vi "Redetection_Baseline calculation.vi"(6 "Sweep #":i32, 8 "File Paramters":T2, 9 "Sweep trace (1D)":cluster{"Ramp Pattern":dbl[], "X":dbl[]}[](array[cluster]), 10 "Detected event":cluster{dbl[][]}, 11 "Data type":T4 items=["AXON", "HEKA"]) -> (3 "New baseline info":cluster{dbl[][]})   [LabVIEW 2017]
uses:
  Data type_new.ctl
  Baseline selection.ctl
  <vilib>/Analysis/baseanly.llb/Mean (DBL).vi
  <vilib>/Analysis/NI_AALBase.lvlib
  <vilib>/Analysis/NI_AALPro.lvlib
panel:
  out "Baseline":cluster{T1[], dbl[]}
  out "XY 그래프":cluster{dbl[], dbl[]}[](graph)
  out "Histogram Graph":T3(graph) caption="히스토그램 그래프"
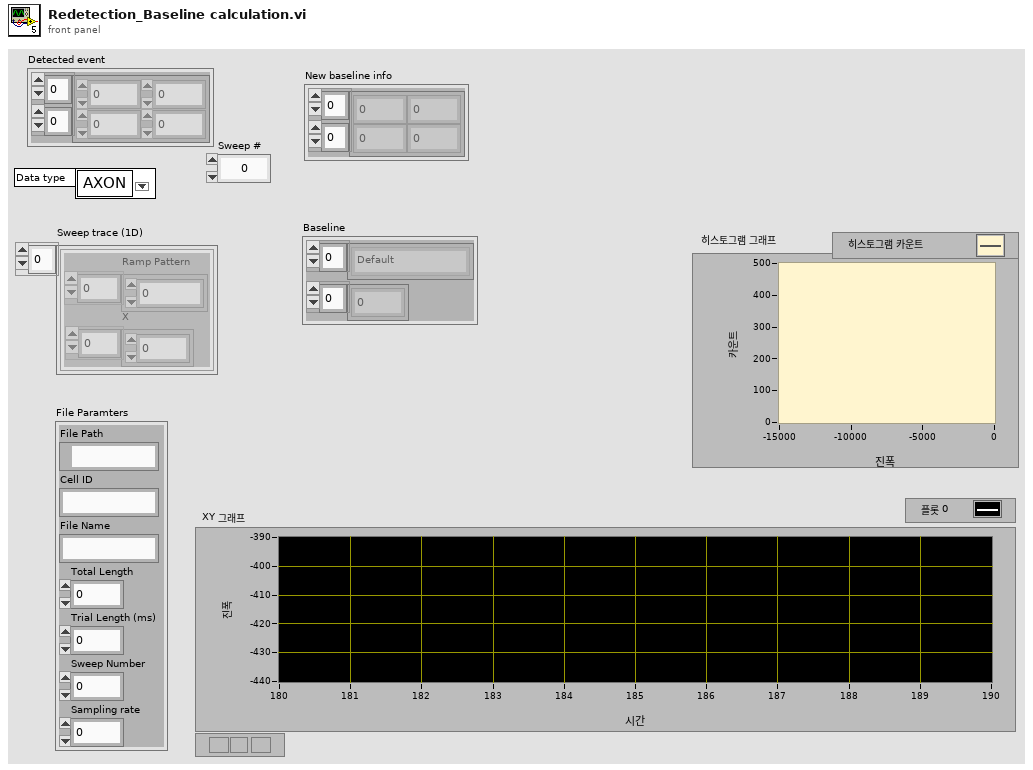
[diagram p1: front panel]
types:
  T1 = typedef "Baseline selection.ctl" = enum16{"Default", "Manual"}
  T2 = cluster{"File Path":path, "Cell ID":string, "File Name":string, "Total Length":i32, "Trial Length (ms)":dbl, "Sweep Number":dbl, "Sampling rate":dbl}
  T3 = cluster{"X Values":dbl[], "Histogram: h(x)":i32[]}
  T4 = typedef "Data type_new.ctl" = u16
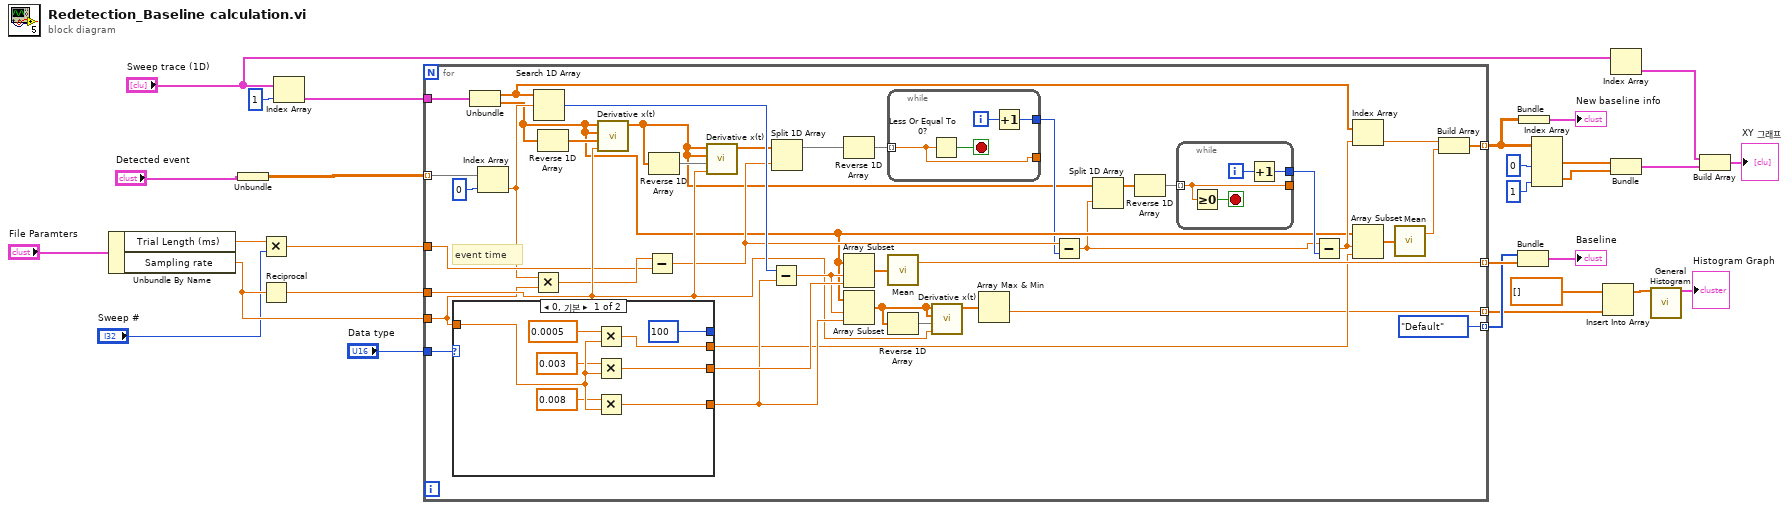
[diagram p0: block diagram]
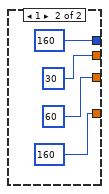
[diagram p2: hidden frame]
diagram:
  n1 = Unbundle By Name("File Paramters") -> ("Trial Length (ms)"=w18:dbl, "Sampling rate"=w4:dbl)
  n2 = Unbundle("Detected event") -> (w1:dbl[][])
  n3 = Multiply(x=w18, y="Sweep #") -> (x*y=w5:dbl)
  n4 = Reciprocal(x=w4) -> (1/x=w11:dbl)
  n5 = Index Array(array="Sweep trace (1D)", index=1 ("인덱스")) -> (element=w15:cluster{"Ramp Pattern":dbl[], "X":dbl[]})
  n6 = for {
    tunnel: w15 -> [w41]
    tunnel: w1 -> [w43] mode=indexing
    tunnel: [w66] -> w14 mode=indexing
    tunnel: "Data type" -> [w68]
    tunnel: [Baseline_selection."Default" ("Baseline selection")] -> w13 mode=indexing
    tunnel: w11 -> [w40]
    tunnel: [w53] -> w10 mode=indexing
    tunnel: [w52] -> w12 mode=indexing
    tunnel: w4 -> [w35]
    tunnel: w5 -> [w38]
    # "event time"
    n7 = case shown="0, 기본" w68 {
      tunnel: [w78 160 ("y")] -> w56
      tunnel: [100 ("길이") 160 ("길이")] -> _
      tunnel: [w79 60 ("길이")] -> w65
      tunnel: [w77 30 ("길이")] -> w55
      tunnel: w35 -> [w83 _]
      frame 0, Default {
        n8 = Multiply(x=0.0005, y=w83) -> (x*y=w77:dbl)
        n9 = Multiply(x=0.003, y=w83) -> (x*y=w79:dbl)
        n10 = Multiply(x=0.008, y=w83) -> (x*y=w78:dbl)
      }
      frame 1 {
      }
    }
    n11 = Unbundle(w41) -> ("Ramp Pattern"=w37:dbl[], "X"=w33:dbl[])
    n12 = Index Array(array=w43, index=0 ("인덱스")) -> (element=w36:dbl)
    n13 = Multiply(x=w36, y=w35) -> (x*y=w39:dbl)
    n14 = Search 1D Array(1D array=w37, element=w36) -> (index of element=w63:i32)  [unwired: 1 in]
    n15 = Reverse 1D Array(array=w33) -> (reversed array=w49:dbl[])
    n16 = call <vilib>:"Derivative x(t).vi"("dt"=w40, "Final Condition"=w49, "Initial Condition"=w33, "X"=w33) -> ("dX/dt"=w29:dbl[])  [unwired: 6 in, 1 out]
    n17 = Subtract(x=w39, y=w38) -> (x-y=w34:dbl)
    n18 = Reverse 1D Array(array=w29) -> (reversed array=w48:dbl[])
    n19 = call <vilib>:"Derivative x(t).vi"("dt"=w40, "Final Condition"=w48, "Initial Condition"=w29, "X"=w29) -> ("dX/dt"=w32:dbl[])  [unwired: 6 in, 1 out]
    n20 = Subtract(x=w63, y=w56) -> (x-y=w54:dbl)
    n21 = Split 1D Array(array=w32, index=w34) -> (first subarray=w47:dbl[])  [unwired: 1 out]
    n22 = Reverse 1D Array(array=w47) -> (reversed array=w46:dbl[])
    n23 = Array Subset(array=w33, index=w54, length=w65) -> (w64:dbl[])
    n24 = Array Subset(array=w33, index=w54, length=w56) -> (w62:dbl[])
    n25 = while {
      tunnel: w46 -> [w71] mode=indexing
      tunnel: [w71] -> _
      tunnel: [w69] -> w31
      i -> [w70]
      stop <- w72 stop-if-true
      n26 = Less Or Equal To 0?(x=w71) -> (x <= 0?=w72:bool)
      n27 = Increment(x=w70) -> (x+1=w69:i32)
    }
    n28 = call-poly <vilib>:"Mean.vi"("X"=w64) -> ("mean"=w66:dbl)  [unwired: 1 out]
    n29 = Reverse 1D Array(array=w62) -> (reversed array=w57:dbl[])
    n30 = call <vilib>:"Derivative x(t).vi"("dt"=w40, "Final Condition"=w57, "Initial Condition"=w62, "X"=w62) -> ("dX/dt"=w51:dbl[])  [unwired: 6 in, 1 out]
    n31 = Array Max & Min(array=w51) -> (min value=w52:dbl)  [unwired: 3 out]
    n32 = Subtract(x=w34, y=w31) -> (x-y=w30:dbl)
    n33 = Split 1D Array(array=w29, index=w30) -> (first subarray=w50:dbl[])  [unwired: 1 out]
    n34 = Reverse 1D Array(array=w50) -> (reversed array=w58:dbl[])
    n35 = while {
      tunnel: w58 -> [w75] mode=indexing
      tunnel: [w75] -> _
      tunnel: [w73] -> w45
      i -> [w74]
      stop <- w76 stop-if-true
      n36 = Greater Or Equal To 0?(x=w75) -> (x >= 0?=w76:bool)
      n37 = Increment(x=w74) -> (x+1=w73:i32)
    }
    n38 = Subtract(x=w30, y=w45) -> (x-y=w44:dbl)
    n39 = Index Array(array=w37, index=w44) -> (element=w59:dbl)
    n40 = Array Subset(array=w33, index=w44, length=w55) -> (w60:dbl[])
    n41 = call-poly <vilib>:"Mean.vi"("X"=w60) -> ("mean"=w61:dbl)  [unwired: 1 out]
    n42 = Build Array(w59, w61) -> (w53:dbl[])
  }
  n43 = Bundle(w13, w14) -> (→"Baseline":cluster{T1[], dbl[]})  [unwired: 1 in]
  n44 = Bundle(w10) -> (→"New baseline info":cluster{dbl[][]})  [unwired: 1 in]
  n45 = Index Array(array=w10, index (col) #1=0 ("비활성화된 인덱스 (열)"), index (col) #2=1 ("인덱스 (열)")) -> (element #1=w9:dbl[], element #2=w8:dbl[])  [unwired: 2 in]
  n46 = Insert Into Array(array=dbl[] [], new element=w12) -> (w24:dbl[])  [unwired: 1 in]
  n47 = Index Array(array="Sweep trace (1D)") -> (element=w21:cluster{"Ramp Pattern":dbl[], "X":dbl[]})  [unwired: 1 in]
  n48 = Bundle(w9, w8) -> (w22:cluster{dbl[], dbl[]})  [unwired: 1 in]
  n49 = call <vilib>:"General Histogram.vi"("X"=w24) -> ("Histogram Graph"=→"Histogram Graph":T3)  [unwired: 10 in, 4 out]
  n50 = Build Array(w21, w22) -> (→"XY 그래프":cluster{"Ramp Pattern":dbl[], "X":dbl[]}[])
